vi "Ic distribution Contour_KeiField.vi"() -> ()   [LabVIEW 2017]
uses:
  <vilib>/Utility/file.llb/Write Delimited Spreadsheet (DBL).vi
  global.vi
panel:
  in  "Scale factor":dbl=1.715265866209262
  out "Current Field mT":dbl=0.8662092624356774
  in  "Step Ramp Time s":dbl=1.0
  in  "Init Ramp Time s":dbl=250.0
  in  "Frequency Hz":dbl=50.0
  in  "Vmax":dbl=2.0
  out "Current Field V":dbl=0.5050000000000001
  in  "KEITHLEY 2400 GPIB Address":string="22"
  out "error out":errorcluster
  in  "Name":string="book13"
  in  "Contour plot folder":path=path "\\\\ad.uillinois.edu\\engr/mrl-dvh-research/Guang Yue/data/Contour plot"
  in  "End field V":dbl=2.0 format="%#_13g"
  in  "Field step V":dbl=0.01 format="%#_13g"
  in  "Start field V":dbl=-3.5 format="%#_13g"
  # "Set default of Ic VI before Run."
  # "V_Field*Scale=mT"
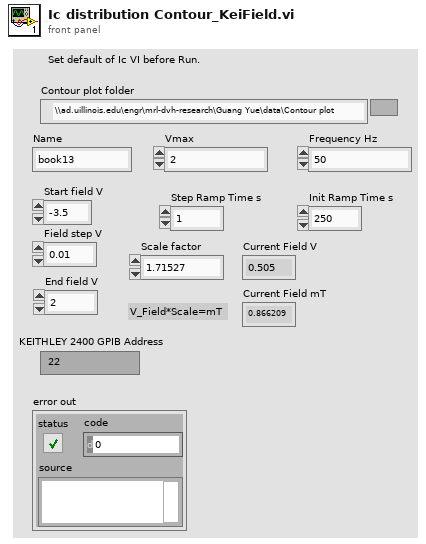
[diagram p1: front panel]
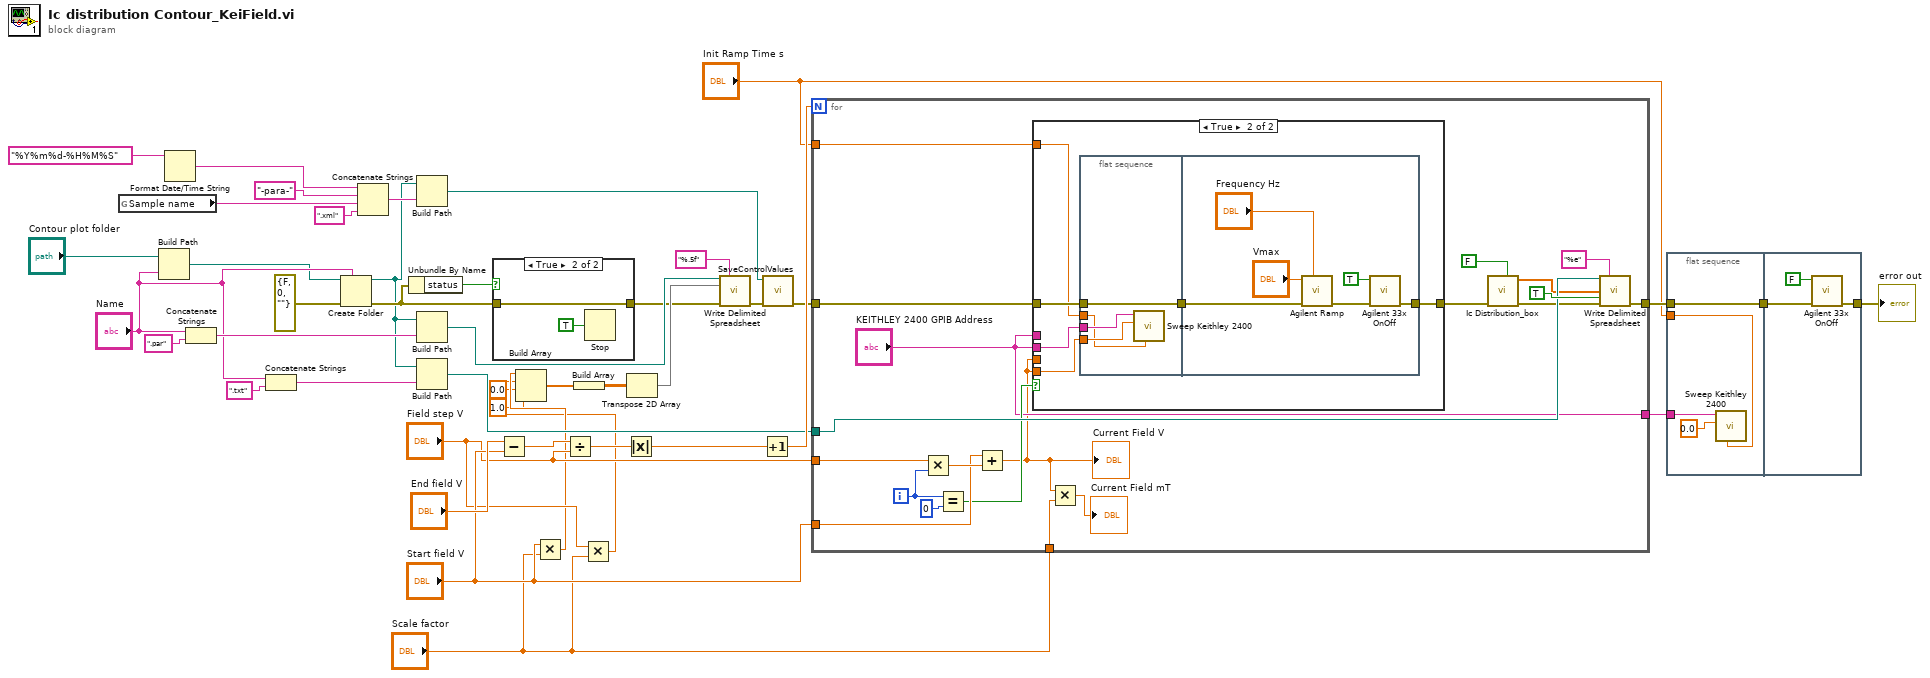
[diagram p0: block diagram]
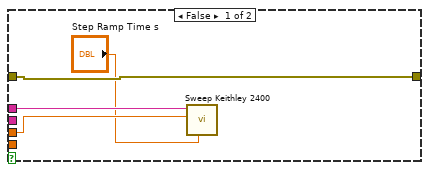
[diagram p3: hidden frame]
diagram:
  n1 = global read "global.vi" "Sample name"() -> (w14:string)
  n2 = Build Path(base path="Contour plot folder", name or relative path="Name") -> (appended path=w21:path)
  n3 = Format Date/Time String(time format string (%c)="%Y%m%d-%H%M%S") -> (date/time string=w15:string)  [unwired: 2 in]
  n4 = Concatenate Strings("Name", ".par" ("string")) -> (w32:string)
  n5 = Concatenate Strings("Name", ".txt" ("string")) -> (w25:string)
  n6 = Create Folder(prompt (Create Folder)="Name", path (use dialog)=w21, error in=errorcluster {"status"=FALSE, "code"=0, "source"=""}) -> (created path=w16:path, error out=w18:errorcluster)  [unwired: 1 out]
  n7 = Concatenate Strings(w15, "-para-" ("string"), w14, ".xml" ("string")) -> (w36:string)
  n8 = Unbundle By Name(w18) -> ("status"=w19:bool)
  n9 = Build Path(base path=w16, name or relative path=w36) -> (appended path=w34:path)
  n10 = Build Path(base path=w16, name or relative path=w32) -> (appended path=w31:path)
  n11 = Build Path(base path=w16, name or relative path=w25) -> (appended path=w24:path)
  n12 = case shown="True" w19 {
    tunnel: [w45 w47] -> w17
    tunnel: w18 -> [w45 w47]
    frame False {
    }
    frame True {
      n13 = Stop(stop? (T)=TRUE) -> ()
    }
  }
  n14 = Subtract(x="End field V", y="Start field V") -> (x-y=w43:dbl)
  n15 = Multiply(x="Start field V", y="Scale factor") -> (x*y=w4:dbl)
  n16 = Divide(x=w43, y="Field step V") -> (x/y=w42:dbl)
  n17 = Multiply(x="Field step V", y="Scale factor") -> (x*y=w3:dbl)
  n18 = Build Array(w4, w3, 0.0 ("element"), 1.0 ("element")) -> (w29:dbl[])
  n19 = Build Array(w29) -> (w28:dbl[][])
  n20 = Absolute Value(x=w42) -> (abs(x)=w41:dbl)
  n21 = Transpose 2D Array(2D array=w28) -> (transposed array=w27:dbl[][])
  n22 = call-poly <vilib>:"Write Delimited Spreadsheet.vi"("file path (dialog if empty)"=w31, "format (%.3f)"="%.5f", "2D data"=w27, "error in (no error)"=w17) -> ("error out"=w20:errorcluster)  [unwired: 10 in, 1 out]
  n23 = Increment(x=w41) -> (x+1=w40:dbl)
  n24 = call "SaveControlValues.vi"("XML File Path"=w34, "error in (no error)"=w20) -> ("error out"=w13:errorcluster)  [unwired: 8 in]
  n25 = for {
    N: w40 -> [_]
    tunnel: "Start field V" -> [w66]
    tunnel: "Field step V" -> [w65]
    tunnel: w24 -> [w60]
    tunnel: w13 -> [w58]
    tunnel: [w54] -> w12
    tunnel: ["KEITHLEY 2400 GPIB Address"] -> w11
    tunnel: "Init Ramp Time s" -> [w51]
    tunnel: "Scale factor" -> [w48]
    i -> [w64]
    n26 = Multiply(x=w65, y=w64) -> (x*y=w67:dbl)
    n27 = Equal?(x=w64, y=0) -> (x = y?=w59:bool)
    n28 = Add(x=w66, y=w67) -> (x+y=w49:dbl)
    "Current Field V" <- w49
    n29 = case shown="True" w59 {
      tunnel: w49 -> [w70 _]
      tunnel: "KEITHLEY 2400 GPIB Address" -> [w71 _]
      tunnel: w58 -> [w69 w74]
      tunnel: [w69 w73] -> w57
      tunnel: w49 -> [_ w77]
      tunnel: "KEITHLEY 2400 GPIB Address" -> [_ w76]
      tunnel: w51 -> [_ w72]
      frame False {
        n30 = call "Sweep Keithley 2400.vi"("Ramp Time (s)"="Step Ramp Time s", "final gate voltage (V)"=w70, "KEITHLEY 2400 GPIB Address"=w71) -> ()  [unwired: 7 in, 2 out]
      }
      frame True {
        n31 = flat-sequence {
          tunnel: w77 -> [w81]
          tunnel: w76 -> [w80]
          tunnel: [w79] -> w75
          tunnel: w74 -> [w79]
          tunnel: w72 -> [w78]
          tunnel: w75 -> [w87]
          tunnel: [w85] -> w73
          frame #0 {
            n32 = call "Sweep Keithley 2400.vi"("Ramp Time (s)"=w78, "final gate voltage (V)"=w81, "KEITHLEY 2400 GPIB Address"=w80) -> ()  [unwired: 7 in, 2 out]
          }
          frame #1 {
            n33 = call "Agilent Ramp.vi"("Frequency Hz"="Frequency Hz", "error in (no error)"=w87, "Vmax"="Vmax") -> ("error out"=w86:errorcluster)  [unwired: 8 in]
            n34 = call "Agilent 33x OnOff.vi"("error in (no error)"=w86, "Enable Output  (T: Enable)"=TRUE) -> ("error out"=w85:errorcluster)  [unwired: 9 in]
          }
        }
      }
    }
    n35 = Multiply(x=w49, y=w48) -> (x*y=→"Current Field mT":dbl)
    n36 = call "Ic Distribution_box.vi"("Log Data"=FALSE, "error in no error"=w57) -> ("error out"=w55:errorcluster, "Ic array"=w56:dbl[])  [unwired: 8 in]
    n37 = call-poly <vilib>:"Write Delimited Spreadsheet.vi"("file path (dialog if empty)"=w60, "format (%.3f)"="%e", "1D data"=w56, "append to file? (new file:F)"=TRUE ("append to file? (F)"), "error in (no error)"=w55) -> ("error out"=w54:errorcluster)  [unwired: 9 in, 1 out]
  }
  n38 = flat-sequence {
    tunnel: w12 -> [w91]
    tunnel: w11 -> [w89]
    tunnel: [w91] -> w9
    tunnel: "Init Ramp Time s" -> [w88]
    tunnel: [w93] -> w10
    tunnel: w9 -> [w94]
    frame #0 {
      n39 = call "Sweep Keithley 2400.vi"("Ramp Time (s)"=w88, "final gate voltage (V)"=0.0, "KEITHLEY 2400 GPIB Address"=w89) -> ()  [unwired: 7 in, 2 out]
    }
    frame #1 {
      n40 = call "Agilent 33x OnOff.vi"("error in (no error)"=w94, "Enable Output  (T: Enable)"=FALSE) -> ("error out"=w93:errorcluster)  [unwired: 9 in]
    }
  }
  "error out" <- w10
